vi "Write Housekeeping.vi"(8 "error in":errorcluster, 10 "CRDS Data in":refnum<class "CRDS Data.lvclass">, 11 "File Obs in":refnum<class "CRD File Obs.lvclass">) -> (0 "error out":errorcluster, 2 "CRD Data Out":refnum<class "CRDS Data.lvclass">, 3 "File Obs Out":refnum<class "CRD File Obs.lvclass">)   [LabVIEW 2015, in "CRD File Obs.lvclass"]
uses:
  CRD File Obs.lvclass
  Data/Main/CRDS Data.lvclass
  Data/Main/crd_data_enum.ctl
  File IO/Class/File Observer.lvclass/File Observer.ctl
  File IO/Class/Read File Ref.vi
  Data/Main/Read CellData.vi
  Data/Cell/CRDS Cell Data.lvclass
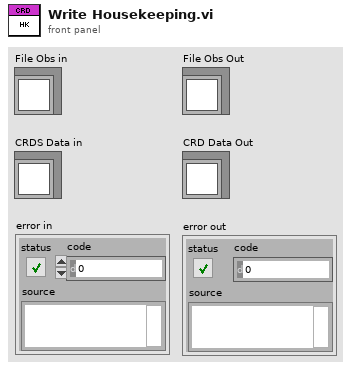
[diagram p1: front panel]
types:
  T1 = enum16{"big-endian, network order", "native, host order", "little-endian"}
  T2 = typedef "crd_data_enum.ctl" = enum8{"Time", "RHw", "TRH", "P", "Tmean", "RHsense", "TQ", "PQ", "Q", "Q0", "Qcal", "Qset", "extDilFac", "taucorr", "tau0corr", "stdevtau", "ext", "extCorr", "etau", "tau", "tau0", "Purge_Data", "NoData", "reserved", "Ttec", "Ang Exp", "Gamma", "filter", "fOverride", "notes", "max amp", "Tthermistor", "RhdilFac", "Psense", "TRHsense_bank", "RHsense_bank", "MFC_Data", "Thum", "ThumSP", "O3 Flow", "Pinlet Flow", "CLAP Flow", "O3 Add Valve", "O2 Valve", "O3 Cal"}
  T3 = typedef "calData.ctl" = cluster{"rhDilFac":sgl, "Q":sgl, "Tmean":sgl, "extDilFac":sgl, "rhCell":sgl, "P":sgl, "T":sgl}
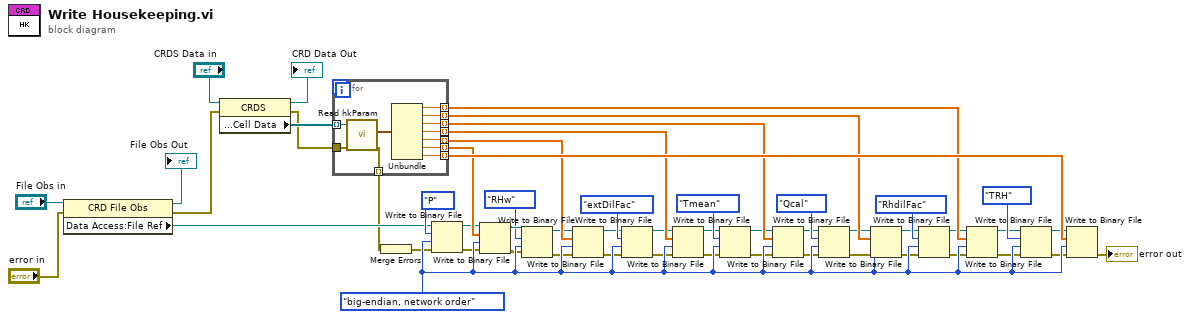
[diagram p0: block diagram]
diagram:
  w52 = T1."big-endian, network order" ("byte order (0:big-endian, network order)")
  n1 = property class="CRD File Obs"(reference="File Obs in", error in="error in") -> (reference out=→"File Obs Out":refnum<class "CRD File Obs.lvclass">, error out=w6:errorcluster, "Data Access:File Ref"=w8:refnum<file>)
  n2 = property class="CRDS"(reference="CRDS Data in", error in=w6) -> (reference out=→"CRD Data Out":refnum<class "CRDS Data.lvclass">, error out=w5:errorcluster, "Data Access:Cell Data"=w10:refnum<class "CRDS Cell Data.lvclass">[])
  n3 = for {
    tunnel: w10 -> [w64] mode=indexing
    tunnel: [w62] -> w43 mode=indexing
    tunnel: [w61] -> w37 mode=indexing
    tunnel: [w60] -> w31 mode=indexing
    tunnel: [w59] -> w25 mode=indexing
    tunnel: [w58] -> w19 mode=indexing
    tunnel: [w57] -> w15 mode=indexing
    tunnel: [w56] -> w51 mode=indexing
    tunnel: w5 -> [w55]
    tunnel: [w54] -> w4 mode=indexing
    n4 = call "Read hkParam.vi"("error in"=w55, "CRDS Cell Data in"=w64) -> ("error out"=w54:errorcluster, "hkParam"=w63:T3)  [unwired: 7 in, 1 out]
    n5 = Unbundle(w63) -> ("rhDilFac"=w62:sgl, "Q"=w61:sgl, "Tmean"=w60:sgl, "extDilFac"=w59:sgl, "rhCell"=w58:sgl, "P"=w57:sgl, "T"=w56:sgl)
  }
  n6 = Merge Errors(w4) -> (w3:errorcluster)
  n7 = Write to Binary File(file (use dialog)=w8, data=crd_data_enum."P" ("CRD_Data_Enum"), error in=w3, 9:w52) -> (refnum out=w12:refnum<file>, error out=w13:errorcluster)  [unwired: 2 in, 1 out]
  n8 = Write to Binary File(file (use dialog)=w12, data=w15, error in=w13, 9:w52) -> (refnum out=w44:refnum<file>, error out=w45:errorcluster)  [unwired: 2 in, 1 out]
  n9 = Write to Binary File(file (use dialog)=w44, data=crd_data_enum."RHw" ("CRD_Data_Enum"), error in=w45, 9:w52) -> (refnum out=w17:refnum<file>, error out=w18:errorcluster)  [unwired: 2 in, 1 out]
  n10 = Write to Binary File(file (use dialog)=w17, data=w19, error in=w18, 9:w52) -> (refnum out=w20:refnum<file>, error out=w21:errorcluster)  [unwired: 2 in, 1 out]
  n11 = Write to Binary File(file (use dialog)=w20, data=crd_data_enum."extDilFac" ("CRD_Data_Enum"), error in=w21, 9:w52) -> (refnum out=w24:refnum<file>, error out=w23:errorcluster)  [unwired: 2 in, 1 out]
  n12 = Write to Binary File(file (use dialog)=w24, data=w25, error in=w23, 9:w52) -> (refnum out=w26:refnum<file>, error out=w27:errorcluster)  [unwired: 2 in, 1 out]
  n13 = Write to Binary File(file (use dialog)=w26, data=crd_data_enum."Tmean" ("CRD_Data_Enum"), error in=w27, 9:w52) -> (refnum out=w29:refnum<file>, error out=w30:errorcluster)  [unwired: 2 in, 1 out]
  n14 = Write to Binary File(file (use dialog)=w29, data=w31, error in=w30, 9:w52) -> (refnum out=w32:refnum<file>, error out=w33:errorcluster)  [unwired: 2 in, 1 out]
  n15 = Write to Binary File(file (use dialog)=w32, data=crd_data_enum."Qcal" ("CRD_Data_Enum"), error in=w33, 9:w52) -> (refnum out=w35:refnum<file>, error out=w36:errorcluster)  [unwired: 2 in, 1 out]
  n16 = Write to Binary File(file (use dialog)=w35, data=w37, error in=w36, 9:w52) -> (refnum out=w39:refnum<file>, error out=w38:errorcluster)  [unwired: 2 in, 1 out]
  n17 = Write to Binary File(file (use dialog)=w39, data=crd_data_enum."RhdilFac" ("CRD_Data_Enum"), error in=w38, 9:w52) -> (refnum out=w41:refnum<file>, error out=w42:errorcluster)  [unwired: 2 in, 1 out]
  n18 = Write to Binary File(file (use dialog)=w41, data=w43, error in=w42, 9:w52) -> (refnum out=w47:refnum<file>, error out=w46:errorcluster)  [unwired: 2 in, 1 out]
  n19 = Write to Binary File(file (use dialog)=w47, data=crd_data_enum."TRH" ("CRD_Data_Enum"), error in=w46, 9:w52) -> (refnum out=w49:refnum<file>, error out=w50:errorcluster)  [unwired: 2 in, 1 out]
  n20 = Write to Binary File(file (use dialog)=w49, data=w51, error in=w50, 9:w52) -> (error out=→"error out":errorcluster)  [unwired: 2 in, 2 out]
